vi "Singl_Qubit_Multpl.vi"(6 "Control Bitmask":bool[][](array[boolean]), 8 "error in (no error)":errorcluster, 9 "2x2 Unitary Matrix":cdb[][](array[numeric]), 10 "QuWire in":refnum<class "QuWire.lvclass">, 11 "SimAlg in":refnum<class "PrllPerElmnt.lvclass">) -> (0 "error out":errorcluster, 2 "QuWire out":refnum<class "QuWire.lvclass">, 3 "SimAlg out":refnum<class "PrllPerElmnt.lvclass">)   [LabVIEW 2020, in "PrllPerElmnt.lvclass"]
uses:
  PrllPerElmnt.lvclass
  QuWire/QuWire.lvclass
  PrllPerElmnt.lvclass/PrllPerElmnt.ctl
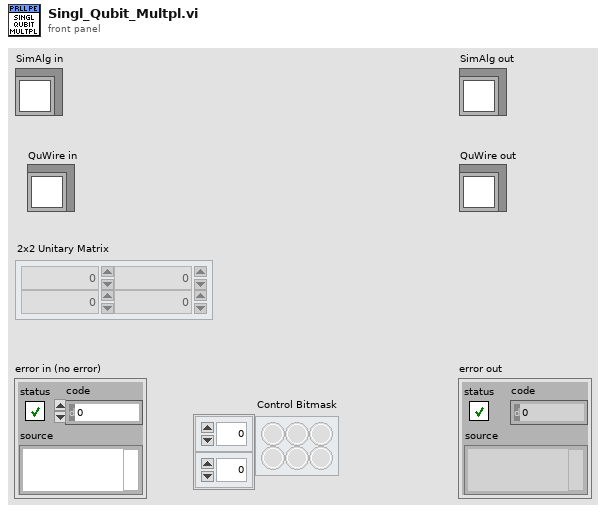
[diagram p1: front panel]
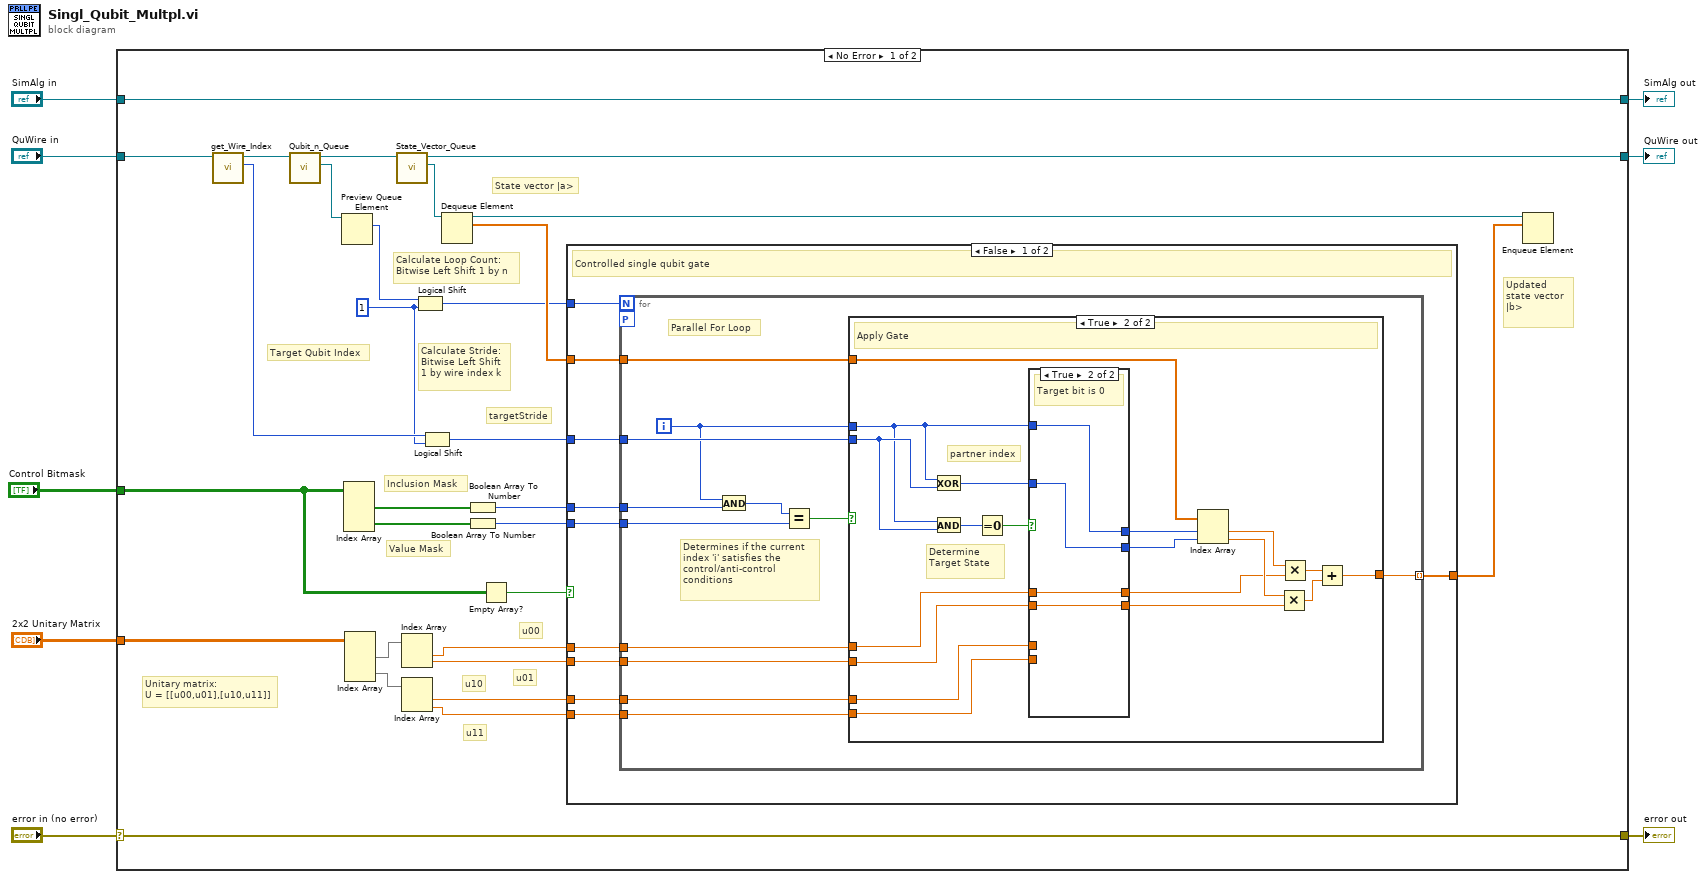
[diagram p0: block diagram]
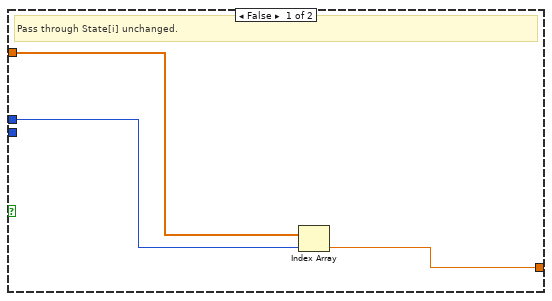
[diagram p2: hidden frame]
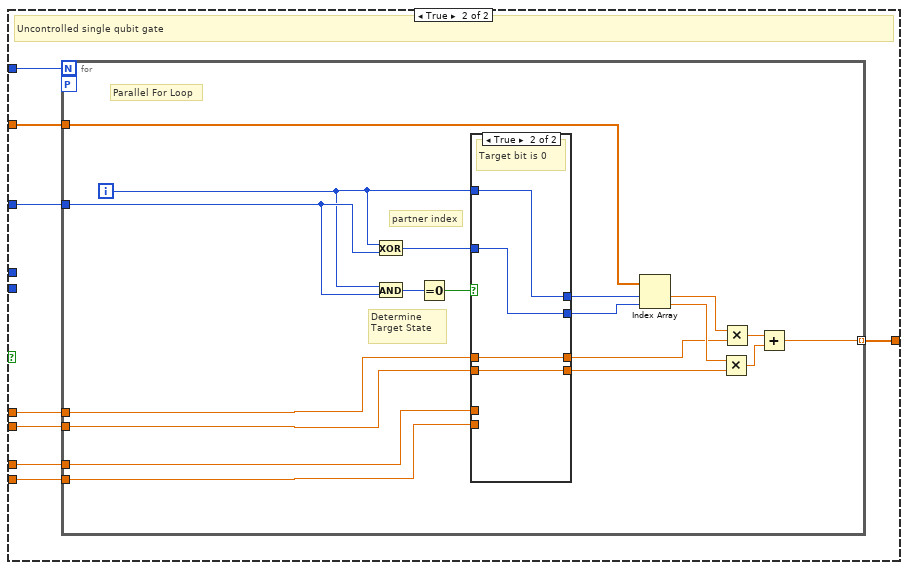
[diagram p4: hidden frame]
diagram:
  n1 = case shown="No Error" "error in (no error)" {
    selector: "error in (no error)" -> [w36 w127]
    tunnel: [w36 w127] -> w7
    tunnel: [w37 w126] -> w5
    tunnel: "SimAlg in" -> [w37 w126]
    tunnel: [w12 w125] -> w4
    tunnel: "QuWire in" -> [w9 w125]
    tunnel: "2x2 Unitary Matrix" -> [w11 _]
    tunnel: "Control Bitmask" -> [w10 _]
    frame No Error {
      w24 = 1 ("x")
      # "targetStride"
      # "Target Qubit Index"
      # "Unitary matrix:\nU = [[u00,u01],[u10,u11]]"
      # "u11"
      # "u10"
      # "u01"
      # "u00"
      # "Updated state vector |b>"
      # "State vector |a>"
      # "Calculate Loop Count: \nBitwise Left Shift 1 by n"
      # "Calculate Stride: \nBitwise Left Shift 1 by wire index k"
      # "Value Mask"
      # "Inclusion Mask"
      n2 = call "get_Wire_Index.vi"("QuWire in"=w9) -> ("Wire Index"=w25:i32, "QuWire out"=w26:refnum<class "QuWire.lvclass">)  [unwired: 8 in, 1 out]
      n3 = call "Qubit_n_Queue.vi"("QuWire in"=w26) -> ("Qubit n"=w27:refnum<queue>, "QuWire out"=w29:refnum<class "QuWire.lvclass">)  [unwired: 8 in, 1 out]
      n4 = Preview Queue Element(queue=w27) -> (element=w28:i32)  [unwired: 2 in, 3 out]
      n5 = Index Array(array=w10) -> (element #1=w23:bool[], element #2=w22:bool[])  [unwired: 4 in]
      n6 = Index Array(array=w11) -> (element #1=w19:cdb[], element #2=w20:cdb[])  [unwired: 4 in]
      n7 = call "State_Vector_Queue.vi"("QuWire in"=w29) -> ("State Vector Queue"=w30:refnum<queue>, "QuWire out"=w12:refnum<class "QuWire.lvclass">)  [unwired: 8 in, 1 out]
      n8 = Index Array(array=w19) -> (element #1=w18:cdb, element #2=w17:cdb)  [unwired: 2 in]
      n9 = Index Array(array=w20) -> (element #1=w14:cdb, element #2=w13:cdb)  [unwired: 2 in]
      n10 = Logical Shift(y=w28, x=w24) -> (x << y=w16:i32)
      n11 = Logical Shift(y=w25, x=w24) -> (x << y=w15:i32)
      n12 = Dequeue Element(queue=w30) -> (queue out=w32:refnum<queue>, element=w31:cdb[])  [unwired: 2 in, 2 out]
      n13 = Boolean Array To Number(Boolean array=w23) -> (number=w21:u32)
      n14 = Boolean Array To Number(Boolean array=w22) -> (number=w34:u32)
      n15 = Empty Array?(array=w10) -> (empty?=w35:bool)
      n16 = case shown="False" w35 {
        tunnel: w13 -> [w47 w97]
        tunnel: w14 -> [w46 w96]
        tunnel: w15 -> [w45 w95]
        tunnel: w16 -> [w44 w94]
        tunnel: w17 -> [w43 w93]
        tunnel: w18 -> [w42 w92]
        tunnel: w34 -> [w41 _]
        tunnel: w21 -> [w40 _]
        tunnel: w31 -> [w39 w91]
        tunnel: [w38 w90] -> w33
        frame False {
          # "Controlled single qubit gate"
          n17 = for {
            N: w44 -> [_]
            tunnel: w40 -> [w52]
            tunnel: w41 -> [w49]
            tunnel: w42 -> [w58]
            tunnel: w43 -> [w57]
            tunnel: w39 -> [w55]
            tunnel: w45 -> [w56]
            tunnel: [w59] -> w38 mode=indexing
            tunnel: w46 -> [w54]
            tunnel: w47 -> [w53]
            workers-P: _ -> [_]
            i -> [w51]
            # "Determines if the current index 'i' satisfies the control/anti-control conditions"
            # "Parallel For Loop"
            n18 = And(x=w51, y=w52) -> (x .and. y?=w50:u32)
            n19 = Equal?(x=w50, y=w49) -> (x = y?=w48:bool)
            n20 = case shown="True" w48 {
              tunnel: [w60 w80] -> w59
              tunnel: w58 -> [_ w76]
              tunnel: w57 -> [_ w75]
              tunnel: w51 -> [w61 w63]
              tunnel: w56 -> [_ w65]
              tunnel: w55 -> [w62 w73]
              tunnel: w54 -> [_ w67]
              tunnel: w53 -> [_ w66]
              frame False {
                # "Pass through State[i] unchanged."
                n21 = Index Array(array=w62, index=w61) -> (element=w60:cdb)
              }
              frame True {
                # "partner index"
                # "Determine Target State"
                # "Apply Gate"
                n22 = Exclusive Or(1:w65, 2:w63) -> (0:w64:i32)
                n23 = And(x=w63, y=w65) -> (x .and. y?=w81:i32)
                n24 = Equal To 0?(x=w81) -> (x = 0?=w77:bool)
                n25 = case shown="True" w77 {
                  tunnel: w76 -> [_ w89]
                  tunnel: w75 -> [_ w88]
                  tunnel: [w83 w87] -> w74
                  tunnel: [w82 w86] -> w70
                  tunnel: [w85 w89] -> w69
                  tunnel: [w84 w88] -> w68
                  tunnel: w67 -> [w85 _]
                  tunnel: w66 -> [w84 _]
                  tunnel: w64 -> [w83 w86]
                  tunnel: w63 -> [w82 w87]
                  frame False {
                    # "Target bit is 1"
                  }
                  frame True {
                    # "Target bit is 0"
                  }
                }
                n26 = Index Array "Index Array"(array=w73, index #1=w74, index #2=w70) -> (element #1=w72:cdb, element #2=w71:cdb)
                n27 = Multiply(x=w71, y=w68) -> (x*y=w79:cdb)
                n28 = Multiply(x=w72, y=w69) -> (x*y=w78:cdb)
                n29 = Add(x=w78, y=w79) -> (x+y=w80:cdb)
              }
            }
          }
        }
        frame True {
          # "Uncontrolled single qubit gate"
          n30 = for {
            N: w94 -> [_]
            tunnel: w92 -> [w115]
            tunnel: w93 -> [w114]
            tunnel: w91 -> [w112]
            tunnel: w95 -> [w113]
            tunnel: [w116] -> w90 mode=indexing
            tunnel: w96 -> [w111]
            tunnel: w97 -> [w110]
            workers-P: _ -> [_]
            i -> [w109]
            # "partner index"
            # "Determine Target State"
            # "Parallel For Loop"
            n31 = Exclusive Or(1:w113, 2:w109) -> (0:w98:i32)
            n32 = And(x=w109, y=w113) -> (x .and. y?=w108:i32)
            n33 = Equal To 0?(x=w108) -> (x = 0?=w105:bool)
            n34 = case shown="True" w105 {
              tunnel: w115 -> [_ w124]
              tunnel: w114 -> [_ w123]
              tunnel: [w118 w122] -> w104
              tunnel: [w117 w121] -> w101
              tunnel: [w120 w124] -> w100
              tunnel: [w119 w123] -> w99
              tunnel: w111 -> [w120 _]
              tunnel: w110 -> [w119 _]
              tunnel: w98 -> [w118 w121]
              tunnel: w109 -> [w117 w122]
              frame False {
                # "Target bit is 1"
              }
              frame True {
                # "Target bit is 0"
              }
            }
            n35 = Index Array "Index Array"(array=w112, index #1=w104, index #2=w101) -> (element #1=w103:cdb, element #2=w102:cdb)
            n36 = Multiply(x=w102, y=w99) -> (x*y=w107:cdb)
            n37 = Multiply(x=w103, y=w100) -> (x*y=w106:cdb)
            n38 = Add(x=w106, y=w107) -> (x+y=w116:cdb)
          }
        }
      }
      n39 = Enqueue Element(queue=w32, element=w33) -> ()  [unwired: 2 in, 3 out]
    }
    frame Error {
    }
  }
  "error out" <- w7
  "SimAlg out" <- w5
  "QuWire out" <- w4
